vi "New DAQ Rack AI Read.vi"(10 "Channel to Cal":T1) -> (0 "Lost Connection":bool, 2 "Available?":bool, 3 "Data":dbl format="%0.2f")   [LabVIEW 2019]
uses:
  Type Defs/New Channel Type Def (RIO).ctl
  Type Defs/TCP Data Stream Mode (PC).ctl
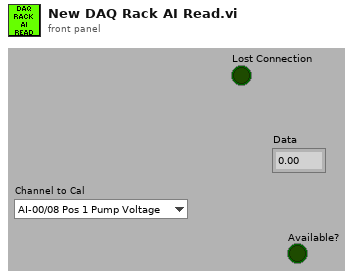
[diagram p1: front panel]
types:
  T1 = typedef "New Channel Type Def (RIO).ctl" = enum16{"AI-00/08 Pos 1 Pump Voltage", "AI-01/09 Pos 2 Pump Voltage", "AI-02/10 Pos 3 Pump Voltage", "AI-03/11 Pos 4 Pump Voltage", "AI-04/12 Pos 5 Pump Voltage", "AI-05/13 Pos 6 Pump Voltage", "AI-06 Spare", "AI-14 Spare", "AI-07 Spare", "AI-15 Power Supply Voltage", "AI-16 Pos 1 Pump Current", "AI-17 Pos 2 Pump Current", "AI-18 Pos 3 Pump Current", "AI-19 Pos 4 Pump Current", "AI-20 Pos 5 Pump Current", "AI-21 Pos 6 Pump Current", "AI-16 Pos 1 Pump Speed", "AI-17 Pos 2 Pump Speed", "AI-18 Pos 3 Pump Speed", "AI-19 Pos 4 Pump Speed", "AI-20 Pos 5 Pump Speed", "AI-21 Pos 6 Pump Speed", "AI-22 Pos 1 Controller Current", "AI-23 Pos 2 Controller Current", "AI-24 Pos 3 Controller Current", "AI-25 Pos 4 Controller Current", "AI-26 Pos 5 Controller Current", "AI-27 Pos 6 Controller Current", "AI-28 Tank 1 Temperature", "AI-29 Tank 2 Temperature", "AI-30 Pos 1 Pump Pressure", "AI-31 Pos 2 Pump Pressure", "AI-32 Pos 3 Pump Pressure", "AI-33 Pos 4 Pump Pressure", "AI-34 Pos 5 Pump Pressure", "AI-35 Pos 6 Pump Pressure", "AI-36 Pos 1 Pump Flow", "AI-37 Pos 2 Pump Flow", "AI-38 Pos 3 Pump Flow", "AI-39 Pos 4 Pump Flow", "AI-40 Pos 5 Pump Flow", "AI-41 Pos 6 Pump Flow", "AI-42 Spare", "AI-43 Spare", "AI-44 Spare", "AI-45 Spare", "AI-46 Spare", "AI-47 Spare", "AI-00/08 Pos 1 Controller Voltage", "AI-01/09 Pos 2 Controller Voltage", "AI-02/10 Pos 3 Controller Voltage", "AI-03/11 Pos 4 Controller Voltage", "AI-04/12 Pos 5 Controller Voltage", "AI-05/13 Pos 6 Controller Voltage"}
  T2 = typedef "TCP Data Stream Mode (PC).ctl" = enum16{"Init", "Read Data", "Close"}
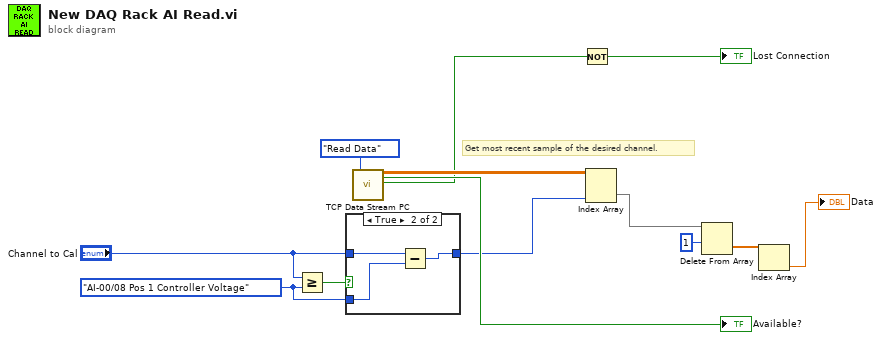
[diagram p0: block diagram]
diagram:
  w8 = New_Channel_Type_Def_(RIO)."AI-00/08 Pos 1 Controller Voltage" ("y")
  # "Get most recent sample of the desired channel."
  n1 = Greater Or Equal?(x="Channel to Cal", y=w8) -> (x >= y?=w9:bool)
  n2 = case shown="True" w9 {
    tunnel: "Channel to Cal" -> [w14 w17]
    tunnel: [w14 w16] -> w1
    tunnel: w8 -> [_ w15]
    frame False {
    }
    frame True {
      n3 = Subtract(x=w17, y=w15) -> (x-y=w16:u16)
    }
  }
  n4 = call "TCP Data Stream PC.vi"("Mode"=TCP_Data_Stream_Mode_(PC)."Read Data") -> ("Data OUT"=w10:dbl[][], "New Data?"=→"Available?":bool, "Connected?"=w7:bool)  [unwired: 15 in, 1 out]
  n5 = Not(x=w7) -> (.not. x?=→"Lost Connection":bool)
  n6 = Index Array(array=w10, index (col)=w1) -> (element=w3:dbl[])  [unwired: 1 in]
  n7 = Delete From Array(array=w3, length=1) -> (deleted portion=w5:dbl[])  [unwired: 1 in, 1 out]
  n8 = Index Array(array=w5) -> (element=→"Data":dbl)  [unwired: 1 in]
